vi "To output format.vi"(8 "input valid":bool=TRUE, 10 "factor":u16, 11 "Data in":fxp<+/-,32,14>[](array[numeric])=[0.0, 0.0]) -> (0 "output valid":bool, 3 "Data out":fxp<+/-,16,14>[](array[numeric]))   [LabVIEW 2018]
uses:
  <vilib>/rvi/FXPMathLib/FxpConvert/subVIs/nifxpmath_Convert_SimConfig.ctl
  <vilib>/fxp/LVFixedPointQuantizationPolicyTypeDef.ctl
  <vilib>/fxp/LVFixedPointOverflowPolicyTypeDef.ctl
  <vilib>/rvi/FXPMathLib/FxpConvert/simVIs/DllFxpConvertTemp_sub.vi
  <vilib>/rvi/FXPMathLib/FxpInterpret/XNode/nifxpmath_Interpret.xnode
  <vilib>/rvi/FXPMathLib/FxpConvert/XNode/nifxpmath_Convert.xnode
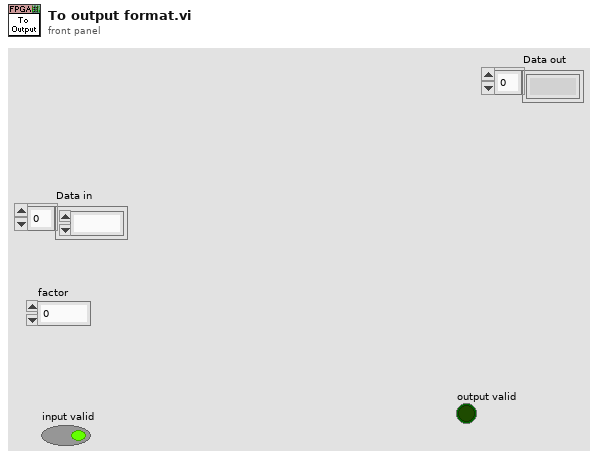
[diagram p1: front panel]
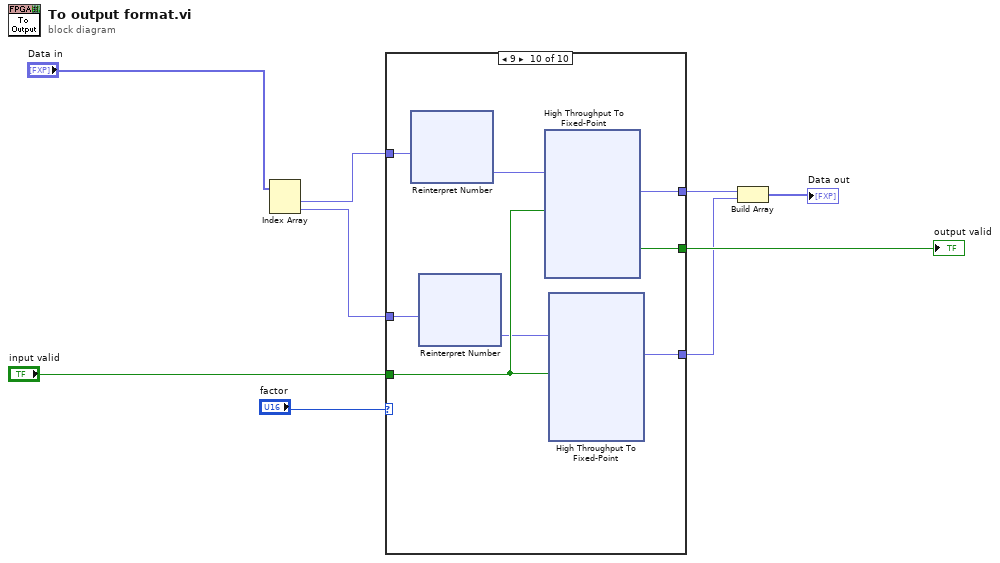
[diagram p0: block diagram]
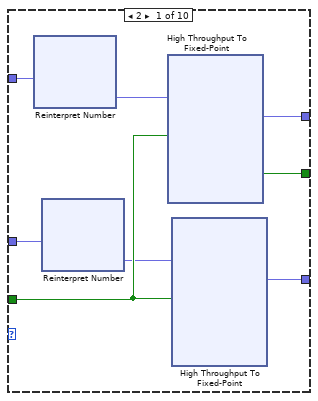
[diagram p2: hidden frame]
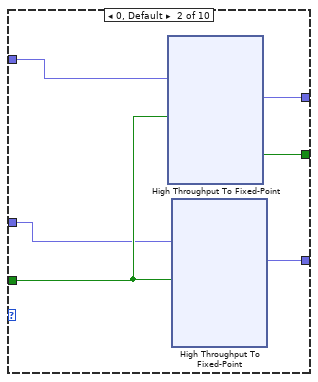
[diagram p3: hidden frame]
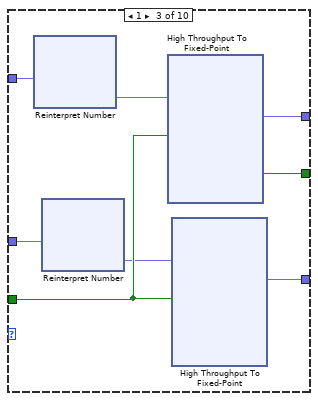
[diagram p4: hidden frame]
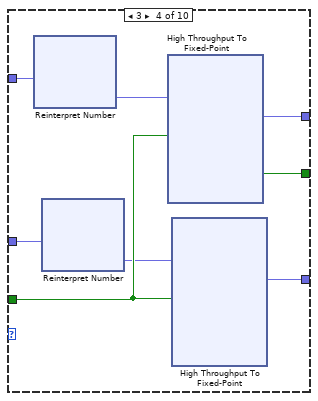
[diagram p5: hidden frame]
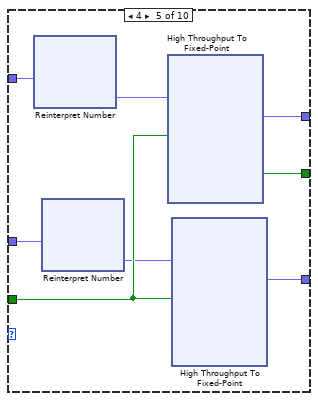
[diagram p6: hidden frame]
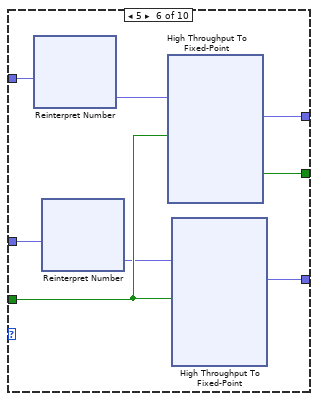
[diagram p7: hidden frame]
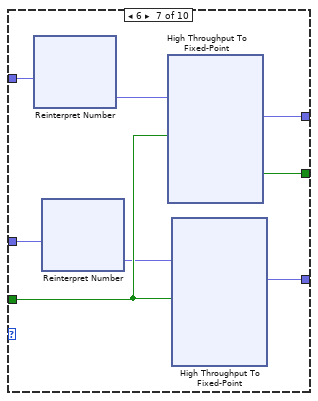
[diagram p8: hidden frame]
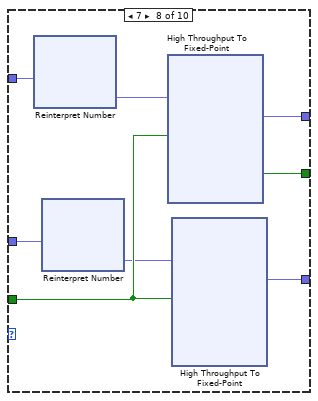
[diagram p9: hidden frame]
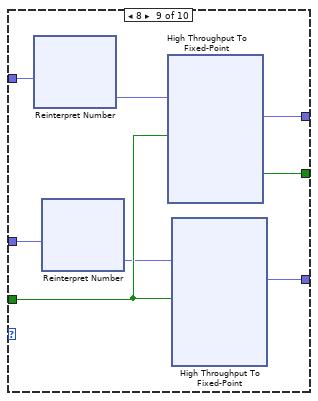
[diagram p10: hidden frame]
diagram:
  n1 = Index Array(array="Data in") -> (element #1=w3:fxp<+/-,32,14>, element #2=w2:fxp<+/-,32,14>)  [unwired: 2 in]
  n2 = case shown="9" "factor" {
    tunnel: "input valid" -> [w17 w71 w127 w183 w239 w295 w351 w407 w463 w519]
    tunnel: [w16 w70 w126 w182 w238 w294 w350 w406 w462 w518] -> w8
    tunnel: [w15 w69 w125 w181 w237 w293 w349 w405 w461 w517] -> w7
    tunnel: [w14 w68 w124 w180 w236 w292 w348 w404 w460 w516] -> w6
    tunnel: w3 -> [w13 w67 w123 w179 w235 w291 w347 w403 w459 w515]
    tunnel: w2 -> [w11 w66 w121 w177 w233 w289 w345 w401 w457 w513]
    frame 2 {
      n3 = xnode "Reinterpret Number"("x"=w13) -> ("y"=w12:fxp<+/-,32,16>)
      n4 = xnode "Reinterpret Number"("x"=w11) -> ("y"=w10:fxp<+/-,32,16>)
      n5 = xnode "High Throughput To Fixed-Point"("x"=w12, "input valid"=w17) -> ("y"=w15:fxp<+/-,16,14>, "output valid"=w16:bool)  [unwired: 1 in, 1 out]
      n6 = xnode "High Throughput To Fixed-Point"("x"=w10, "input valid"=w17) -> ("y"=w14:fxp<+/-,16,14>)  [unwired: 1 in, 2 out]
    }
    frame 0, Default {
      n7 = xnode "High Throughput To Fixed-Point"("x"=w67, "input valid"=w71) -> ("y"=w69:fxp<+/-,16,14>, "output valid"=w70:bool)  [unwired: 1 in, 1 out]
      n8 = xnode "High Throughput To Fixed-Point"("x"=w66, "input valid"=w71) -> ("y"=w68:fxp<+/-,16,14>)  [unwired: 1 in, 2 out]
    }
    frame 1 {
      n9 = xnode "Reinterpret Number"("x"=w123) -> ("y"=w122:fxp<+/-,32,15>)
      n10 = xnode "Reinterpret Number"("x"=w121) -> ("y"=w120:fxp<+/-,32,15>)
      n11 = xnode "High Throughput To Fixed-Point"("x"=w122, "input valid"=w127) -> ("y"=w125:fxp<+/-,16,14>, "output valid"=w126:bool)  [unwired: 1 in, 1 out]
      n12 = xnode "High Throughput To Fixed-Point"("x"=w120, "input valid"=w127) -> ("y"=w124:fxp<+/-,16,14>)  [unwired: 1 in, 2 out]
    }
    frame 3 {
      n13 = xnode "Reinterpret Number"("x"=w179) -> ("y"=w178:fxp<+/-,32,17>)
      n14 = xnode "Reinterpret Number"("x"=w177) -> ("y"=w176:fxp<+/-,32,17>)
      n15 = xnode "High Throughput To Fixed-Point"("x"=w178, "input valid"=w183) -> ("y"=w181:fxp<+/-,16,14>, "output valid"=w182:bool)  [unwired: 1 in, 1 out]
      n16 = xnode "High Throughput To Fixed-Point"("x"=w176, "input valid"=w183) -> ("y"=w180:fxp<+/-,16,14>)  [unwired: 1 in, 2 out]
    }
    frame 4 {
      n17 = xnode "Reinterpret Number"("x"=w235) -> ("y"=w234:fxp<+/-,32,18>)
      n18 = xnode "Reinterpret Number"("x"=w233) -> ("y"=w232:fxp<+/-,32,18>)
      n19 = xnode "High Throughput To Fixed-Point"("x"=w234, "input valid"=w239) -> ("y"=w237:fxp<+/-,16,14>, "output valid"=w238:bool)  [unwired: 1 in, 1 out]
      n20 = xnode "High Throughput To Fixed-Point"("x"=w232, "input valid"=w239) -> ("y"=w236:fxp<+/-,16,14>)  [unwired: 1 in, 2 out]
    }
    frame 5 {
      n21 = xnode "Reinterpret Number"("x"=w291) -> ("y"=w290:fxp<+/-,32,19>)
      n22 = xnode "Reinterpret Number"("x"=w289) -> ("y"=w288:fxp<+/-,32,19>)
      n23 = xnode "High Throughput To Fixed-Point"("x"=w290, "input valid"=w295) -> ("y"=w293:fxp<+/-,16,14>, "output valid"=w294:bool)  [unwired: 1 in, 1 out]
      n24 = xnode "High Throughput To Fixed-Point"("x"=w288, "input valid"=w295) -> ("y"=w292:fxp<+/-,16,14>)  [unwired: 1 in, 2 out]
    }
    frame 6 {
      n25 = xnode "Reinterpret Number"("x"=w347) -> ("y"=w346:fxp<+/-,32,20>)
      n26 = xnode "Reinterpret Number"("x"=w345) -> ("y"=w344:fxp<+/-,32,20>)
      n27 = xnode "High Throughput To Fixed-Point"("x"=w346, "input valid"=w351) -> ("y"=w349:fxp<+/-,16,14>, "output valid"=w350:bool)  [unwired: 1 in, 1 out]
      n28 = xnode "High Throughput To Fixed-Point"("x"=w344, "input valid"=w351) -> ("y"=w348:fxp<+/-,16,14>)  [unwired: 1 in, 2 out]
    }
    frame 7 {
      n29 = xnode "Reinterpret Number"("x"=w403) -> ("y"=w402:fxp<+/-,32,21>)
      n30 = xnode "Reinterpret Number"("x"=w401) -> ("y"=w400:fxp<+/-,32,21>)
      n31 = xnode "High Throughput To Fixed-Point"("x"=w402, "input valid"=w407) -> ("y"=w405:fxp<+/-,16,14>, "output valid"=w406:bool)  [unwired: 1 in, 1 out]
      n32 = xnode "High Throughput To Fixed-Point"("x"=w400, "input valid"=w407) -> ("y"=w404:fxp<+/-,16,14>)  [unwired: 1 in, 2 out]
    }
    frame 8 {
      n33 = xnode "Reinterpret Number"("x"=w459) -> ("y"=w458:fxp<+/-,32,22>)
      n34 = xnode "Reinterpret Number"("x"=w457) -> ("y"=w456:fxp<+/-,32,22>)
      n35 = xnode "High Throughput To Fixed-Point"("x"=w458, "input valid"=w463) -> ("y"=w461:fxp<+/-,16,14>, "output valid"=w462:bool)  [unwired: 1 in, 1 out]
      n36 = xnode "High Throughput To Fixed-Point"("x"=w456, "input valid"=w463) -> ("y"=w460:fxp<+/-,16,14>)  [unwired: 1 in, 2 out]
    }
    frame 9 {
      n37 = xnode "Reinterpret Number"("x"=w515) -> ("y"=w514:fxp<+/-,32,23>)
      n38 = xnode "Reinterpret Number"("x"=w513) -> ("y"=w512:fxp<+/-,32,23>)
      n39 = xnode "High Throughput To Fixed-Point"("x"=w514, "input valid"=w519) -> ("y"=w517:fxp<+/-,16,14>, "output valid"=w518:bool)  [unwired: 1 in, 1 out]
      n40 = xnode "High Throughput To Fixed-Point"("x"=w512, "input valid"=w519) -> ("y"=w516:fxp<+/-,16,14>)  [unwired: 1 in, 2 out]
    }
  }
  "output valid" <- w8
  n41 = Build Array(w7, w6) -> (→"Data out":fxp<+/-,16,14>[])
